vi "SIMCOMCommunicationTool.vi"(4 "Slot":T1, 6 "Debug":bool=TRUE, 7 "MEID":string, 8 "error in":errorcluster, 9 "DelayTime":u32=100, 10 "通信协议名称":string, 11 "VISA资源名称":refnum<visa-resource-name>="COM26") -> (0 "error out":errorcluster, 1 "ReturnData":string, 2 "反馈结果":bool=TRUE, 3 "字符串数值":bool=TRUE, 5 "CMD":string="发送 重启:AT+CRESET\r反馈:\r\nOK\r\n\r\n")   [LabVIEW 2013]
doc: "本范例根据用户指示，对串口执行读写操作。范例运行时可按下“写入”或“读取”按钮，以及修改“读数”。\n\n设置的串口参数必须匹配连接仪器或设备的参数。本范例中，“读数”参数可指定串口读取的字节数。如端口字节超过指定的字节数，超出部分将不会被读取。如端口字节数少于指定的字节数，将返回超时错误。\n\n本范例可扩展流控制选项以包括XON和XOFF，从而允许用户选择控制字符。同时，用户可启用或禁用中止符。部分设备需要通过终止符确定命令字符串的结束位置。部分设备将发送终止符以说明待读取数据的末端。本范例演示了缓冲区中检测到终止符时，结束“读取”操作或添加终止符至“写入”数据末端的方法。"
uses:
  SystemCode/SysControl/Slot.ctl
  <vilib>/Utility/NIReport.llb/NI_report.lvclass
  C:/Program Files/National Instruments/LabVIEW 2013/examples/Instrument IO/Serial/support/Serial - Settings.ctl
  SourceCode/GlobalValue.vi
  <vilib>/Utility/error.llb/Error Cluster From Error Code.vi
  <vilib>/addons/_office/excel.llb/Excel Get Data ([str]).vi
  <vilib>/Instr/_visa.llb/VISA Configure Serial Port (Instr).vi
  <vilib>/ErrorRing/Error Ring.xnode
  <vilib>/addons/_office/NI_ReportGenerationToolkit.lvlib
  <vilib>/Utility/NIReport.llb/Excel/NI_Excel.lvclass
panel:
  out "Data":string[][](array[string])=[["8986031490021881534", "460036161669975", "2A645416CB435F94", "8006A127", "460036161669975@mycdma.cn", "DB60264368A1D188", "18101891253", "A1000021A59070"], ["8986031490021881535", "460036161669976", "32FA5764D69C76BE", "80FAE4E6", "460036161669976@mycdma.cn", "B3AA1B3D2F0D5593", "18964872399", "A1000021A58D61"], ["", "", "", "", "", "", "", ""], ["", "", "", "", "", "", "", ""], ["", "", "", "", "", "", "", ""], ["", "", "", "", "", "", "", ""], ["", "", "", "", "", "", "", ""], ["", "", "", "", "", "", "", ""], ["", "", "", "", "", "", "", ""], ["", "", "", "", "", "", "", ""], ["", "各位，模块烧号主要是写五码，包括IMSI、AKEY、MEID（ESN）、AN(EVDO USER)、AAA(EVDO PWD)。", "", "", "", "", "", ""], ["", "其中ESN和MEID在模块出厂时已经写入，两者均可通过AT指令读取，但ESN不可更改。", "", "", "", "", "", ""], ["", "经询问及实际测试，上海电信绑定ESN号而广东电信未绑定，意味着上海电信五码烧录到其它模块是不可用的，但广东电信则无此限制。", "", "", "", "", "", ""], ["", "", "", "", "", "", "", ""], ["", "", "", "", "", "", "", ""], ["", "目前已确定跟上海电信合作，后续模块及卡号使用过程中，如遇到模块损坏，则意味着该卡必须销号（除非向电信申请绑定新的ESN），否则烧录到其它模块中是没用的。", "", "", "", "", "", ""]]
  in  "命令列表":u16(ring)=18 items=["查询RTRECF", "设置RTRECF", "查询MEID", "设置MEID", "查询ESN", "设置ESN", "查询AKEY", "设置AKEY", "查询IMSI1", "设置IMSI1", "查询IMSI2", "设置IMSI2", "查询IMSI3", "设置IMSI3", "设置EVDO账号", "设置EVDO密码", "打开音频LOOPBACK", "关闭音频LOOPBACK", "重启", "打开网络", "查询网络状态", "连网测试", "查询CIP", "切换声音通道", "测试登录", "拨号", "挂断", "查询IP", "AT+CSOCKAUTHNV", "AT+CSOCKAUTH", "查询2G信号", "查询3G信号", "H330测试通讯", "H330打开音频回环", "H330关闭音频回环", "H330拨号"]
  out "ConfigPath":string="D:\\导航\\T-BOX\\新建文件夹\\config\\通信协议.xls"
  out "DataType":string="AT+CRESET"
  out "命令":string="AT+CRESET\r"
  out "响应":string="\r\nOK\r\n"
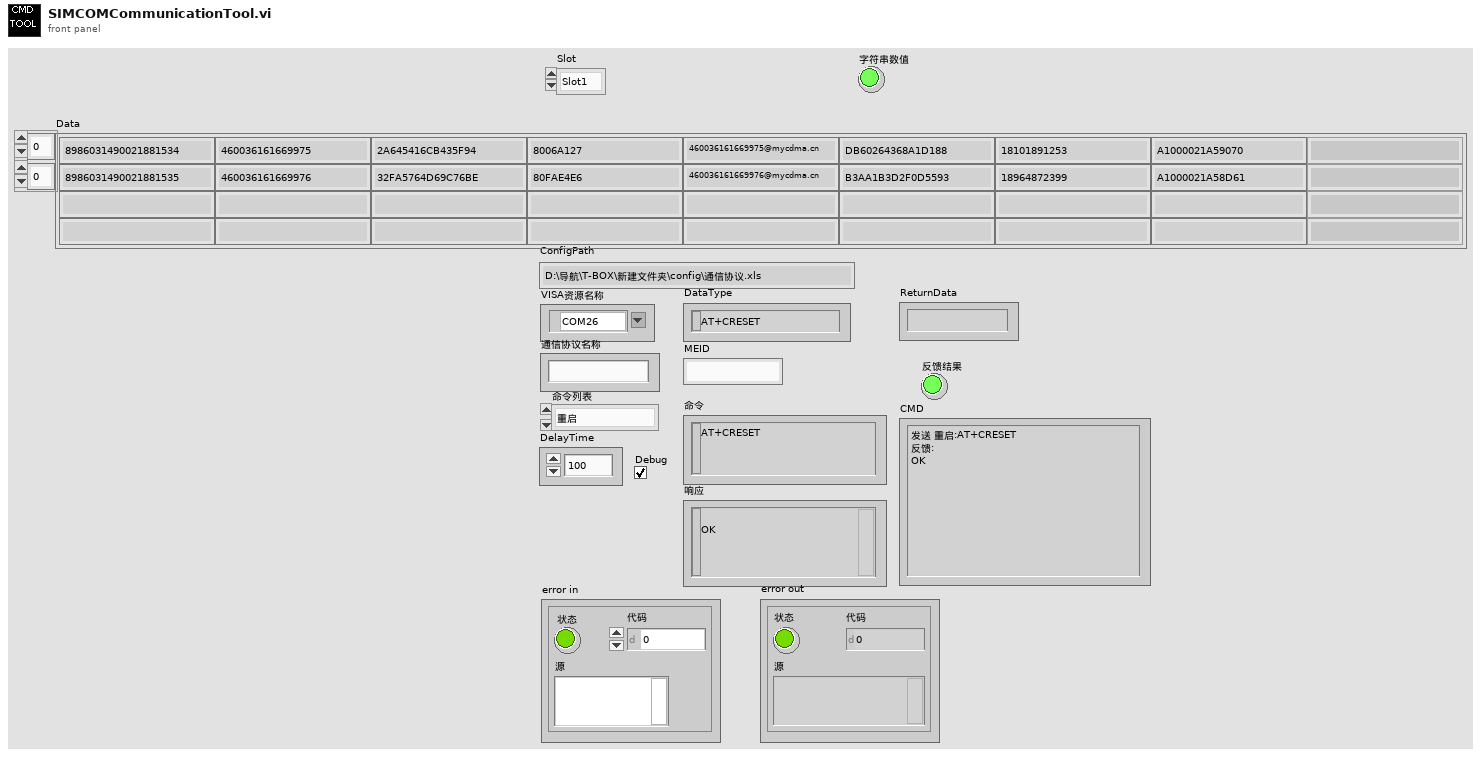
[diagram p1: front panel]
types:
  T1 = typedef "Slot.ctl" = enum16{"Slot1", "Slot2", "Slot3", "Slot4"}
  T2 = enum32{"invalid app kind", "Development System", "Run Time System", "Student Edition", "Embedded LabVIEW", "Evaluation", "Custom"}
  T3 = enum16{"maximized", "minimized", "normal", "no change"}
  T4 = enum16{"Standard Report", "HTML", "Word", "Excel"}
  T5 = typedef "Serial - Settings.ctl" = cluster{"波特率":u32, "数据比特":u16, "奇偶":enum16{"None", "Odd", "Even", "Mark", "Space"}, "停止位":u16, "流控制":u16}
  T6 = cluster{"IMSI":string, "AKEY":string, "ESN":string, "EVDO账号":string, "EVDO密码":string, "设备号":string}
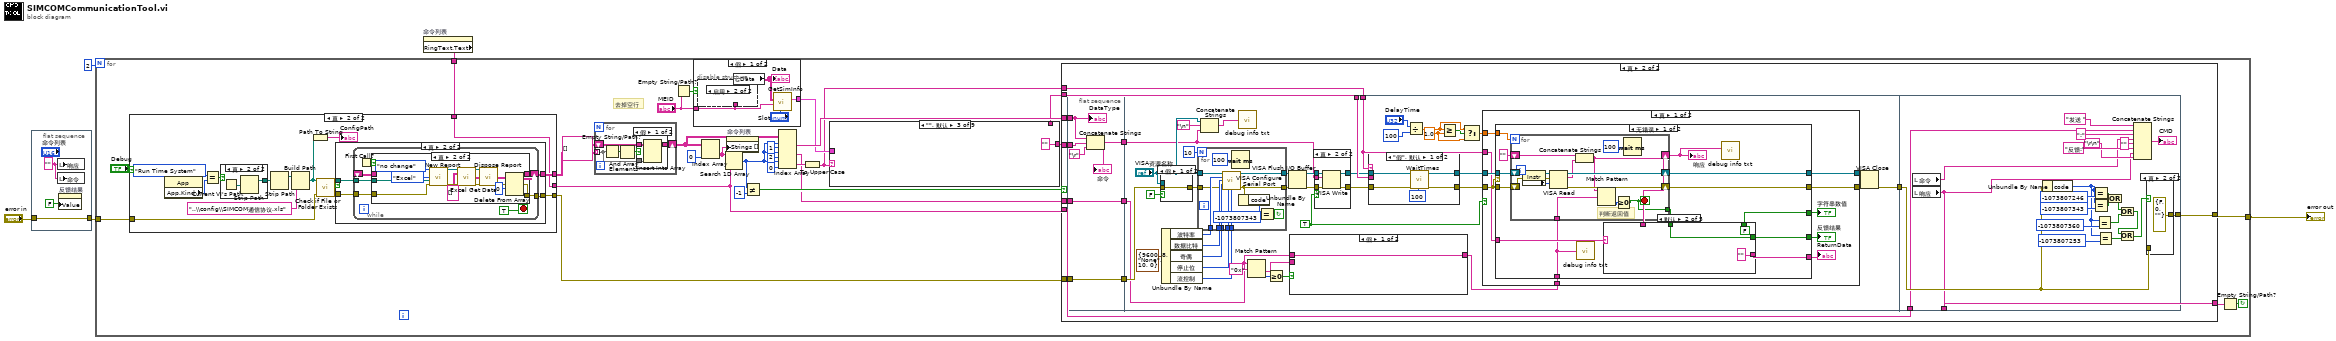
[diagram p0: block diagram]
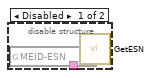
[diagram p2: hidden frame]
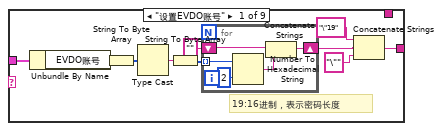
[diagram p5: hidden frame]
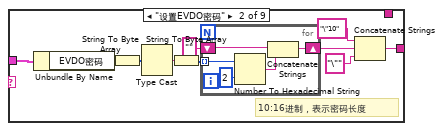
[diagram p6: hidden frame]
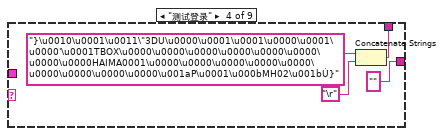
[diagram p7: hidden frame]
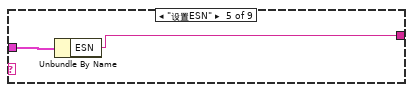
[diagram p8: hidden frame]
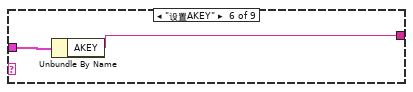
[diagram p9: hidden frame]
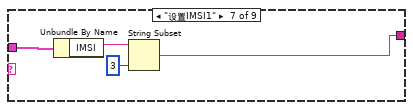
[diagram p10: hidden frame]
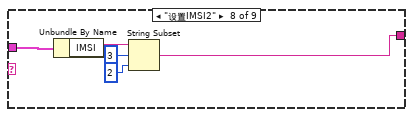
[diagram p11: hidden frame]
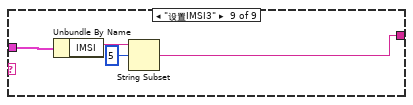
[diagram p12: hidden frame]
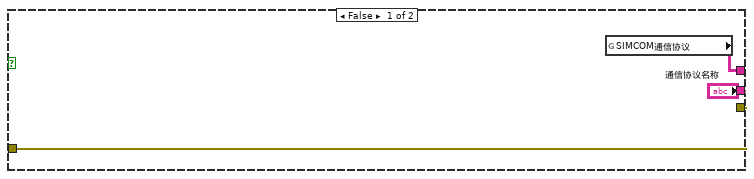
[diagram p13: hidden frame]
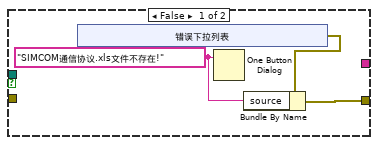
[diagram p14: hidden frame]
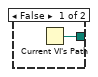
[diagram p16: hidden frame]
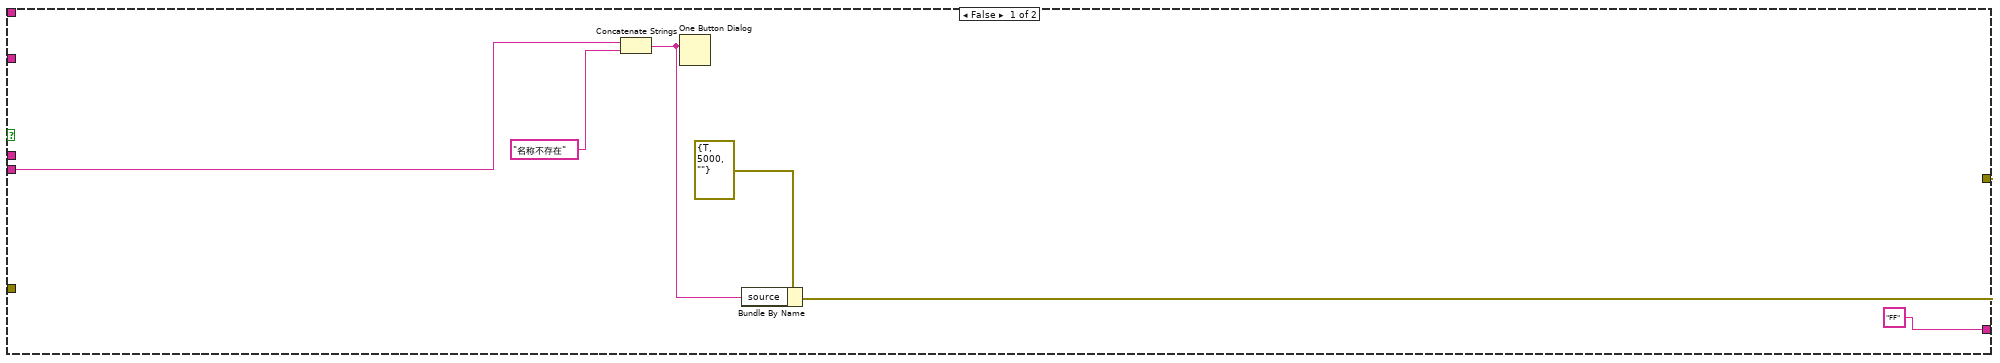
[diagram p17: hidden frame]
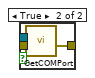
[diagram p18: hidden frame]
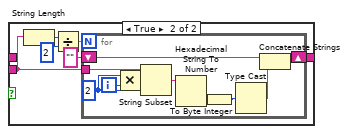
[diagram p19: hidden frame]
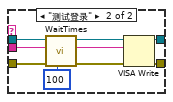
[diagram p20: hidden frame]
diagram:
  n1 = flat-sequence {
    tunnel: "error in" -> [w7]
    tunnel: [w7] -> w2
    frame #0 {
      w8 = "" ("响应")
      n2 = local write "响应"(w8) -> ()
      n3 = local write "命令"(w8) -> ()
      n4 = property on="反馈结果" class="Bool (严格)"("Value"=FALSE ("反馈结果")) -> ()  [unwired: 2 in, 2 out]
    }
  }
  n5 = property on="命令列表" class="Ring (严格)"() -> ("RingText.Text"=w1:string)  [unwired: 2 in, 2 out]
  n6 = for {
    N: 2 -> [_]
    tunnel: w2 -> [w24]
    tunnel: [w36] -> w5
    tunnel: w1 -> [w17]
    stop <- w22 continue-if-true
    # "去掉空行"
    n7 = case shown="真" "Debug" {
      tunnel: [w105 w110] -> w35
      tunnel: w24 -> [w105 w109]
      tunnel: ["通信协议名称" w107] -> w28
      tunnel: [w104 w108] -> w19
      tunnel: w17 -> [_ w107]
      frame False {
        n8 = global read "GlobalValue.vi" "SIMCOM通信协议"() -> (w104:string[][])
      }
      frame True {
        n9 = property class="App"() -> ("App.Kind"=w119:T2)  [unwired: 2 in, 2 out]
        n10 = Equal?(x=T2."Run Time System" ("y"), y=w119) -> (x = y?=w121:bool)
        n11 = case shown="真" w121 {
          tunnel: [w155 w157] -> w120
          frame False {
            n12 = Current VI's Path() -> (path=w155:path)
          }
          frame True {
            n13 = Current VI's Path() -> (path=w156:path)
            n14 = Strip Path(path=w156) -> (stripped path=w157:path)  [unwired: 1 out]
          }
        }
        n15 = Strip Path(path=w120) -> (stripped path=w114:path)  [unwired: 1 out]
        n16 = Build Path(base path=w114, name or relative path="..\\config\\SIMCOM通信协议.xls" ("连接的字符串")) -> (appended path=w116:path)
        n17 = Path To String(path=w116) -> (string=→"ConfigPath":string)
        n18 = call <vilib>:"Check if File or Folder Exists.vi"("error in (no error)"=w109, "path"=w116) -> ("error out"=w111:errorcluster, "file or folder exists?"=w113:bool, "dup path"=w112:path)  [unwired: 7 out]
        n19 = case shown="真" w113 {
          tunnel: w112 -> [_ w132]
          tunnel: w111 -> [_ w131]
          tunnel: [w123 w130] -> w110
          tunnel: [_ w129] -> w108
          frame False {
            w124 = "SIMCOM通信协议.xls文件不存在!" ("消息")
            n20 = xnode "错误下拉列表"() -> ("错误输出"=w122:errorcluster)
            n21 = One Button Dialog(message=w124) -> ()  [unwired: 1 in, 1 out]
            n22 = Bundle By Name(cluster=w122, "source"=w124) -> (w123:errorcluster)
          }
          frame True {
            n23 = while {
              tunnel: w132 -> [w138]
              tunnel: [w137] -> w130
              tunnel: w131 -> [w136]
              shift-right: [w139] -> w129
              shift-left: _ -> [w134]
              stop <- TRUE stop-if-true
              n24 = First Call?() -> (First Call?: T/F=w133:bool)
              n25 = case shown="真" w133 {
                tunnel: [w141 w145] -> w139
                tunnel: w138 -> [_ w144]
                tunnel: [w140 w143] -> w137
                tunnel: w136 -> [w140 w142]
                tunnel: w134 -> [w141 _]
                frame False {
                }
                frame True {
                  n26 = call <vilib>:"New Report.vi"("window state (normal)"=T3."no change", "report type"=T4."Excel", "template (empty)"=w144, "error in (no error)"=w142) -> ("report out"=w150:refnum<class "NI_report.lvclass">, "error out"=w151:errorcluster)  [unwired: 2 in, 8 out]
                  n27 = call-poly <vilib>:"Excel Get Data.vi"("report in"=w150, "data type"=string[][] [], "error in (no error)"=w151) -> ("report out"=w147:refnum<class "NI_report.lvclass">, "data"=w152:string[][], "error out"=w146:errorcluster)  [unwired: 10 in]
                  n28 = call-dynamic "Dispose Report.vi"("report in"=w147, "error in (no error)"=w146) -> ("error out"=w143:errorcluster)  [unwired: 3 in, 10 out]
                  n29 = Delete From Array(array=w152, index (row)=0 ("索引 (行)")) -> (array with subset deleted=w145:string[][])  [unwired: 2 in, 1 out]
                }
              }
            }
          }
        }
      }
    }
    n30 = for {
      tunnel: w19 -> [w43] mode=indexing
      shift-right: [w46] -> w18
      shift-left: string[][] [] -> [w47]
      n31 = Empty String/Path?(string/path=w43) -> (empty?=w45:bool[])
      n32 = And Array Elements(Boolean array=w45) -> (logical AND=w44:bool)
      n33 = case shown="假" w44 {
        tunnel: w47 -> [w50 w51]
        tunnel: [w49 w51] -> w46
        tunnel: w43 -> [w48 _]
        frame False {
          n34 = Insert Into Array(array=w50, new element=w48) -> (w49:string[][])  [unwired: 2 in]
        }
        frame True {
        }
      }
    }
    n35 = Empty String/Path?(string/path="MEID") -> (empty?=w10:bool)
    n36 = case shown="假" w10 {
      tunnel: [w40 _] -> w14
      tunnel: "MEID" -> [w37 _]
      frame False {
        n37 = disable-structure shown="启用" {
          disable-tunnel: w37 -> [w41 _]
          frame Disabled {
            n38 = global read "GlobalValue.vi" "MEID-ESN"() -> (w42:string[][])
            n39 = call "GetESN.vi"("MEID"=w41, "Data"=w42) -> ()  [unwired: 9 in, 1 out]
          }
          frame Enabled {
          }
        }
        n40 = global read "GlobalValue.vi" "Data"() -> (w39:string[][])
        "Data" <- w39
        n41 = call "GetSimInfo.vi"("Slot"="Slot", "MEID"=w37, "Data"=w39) -> ("SIMInfo"=w40:T6)  [unwired: 6 in, 2 out]
      }
      frame True {
      }
    }
    n42 = Index Array(array=w18, index (col)=0 ("禁用的索引 (列)")) -> (element=w26:string[])  [unwired: 1 in]
    n43 = Search 1D Array(1D array=w26, element=w28) -> (index of element=w21:i32)  [unwired: 1 in]
    n44 = property on="命令列表" class="Ring (严格)"("Strings []"=w26) -> ()  [unwired: 2 in, 2 out]
    n45 = Not Equal?(x=w21, y=-1) -> (x != y?=w30:bool)
    n46 = Index Array(array=w18, index (row) #1=w21, index (col) #1=1 ("索引 (列)"), index (row) #2=w21, index (col) #2=2 ("索引 (列)"), index (row) #3=w21, index (col) #3=0 ("索引 (列)")) -> (element #1=w15:string, element #2=w11:string, element #3=w16:string)
    n47 = To Upper Case(1:w16) -> (0:w12:string)
    n48 = case shown="\"\", 默认" w12 {
      tunnel: [w54 w69 "" "" ("IMSI") w87 w89 w91 w96 w101] -> w29
      tunnel: w14 -> [w53 w67 _ _ w88 w90 w94 w99 w103]
      tunnel: [_ _ _ w83 _ _ _ _ _] -> w13
      frame "设置EVDO账号" {
        # "19:16进制，表示密码长度"
        n49 = Unbundle By Name(w53) -> ("EVDO账号"=w52:string)
        n50 = String To Byte Array(string=w52) -> (unsigned byte array=w61:u8[])
        n51 = Type Cast(x=w61) -> (*(type *) &x=w59:string)  [unwired: 1 in]
        n52 = String To Byte Array(string=w59) -> (unsigned byte array=w60:u8[])
        n53 = for {
          tunnel: w60 -> [w66] mode=indexing
          shift-right: [w64] -> w55
          shift-left: "" -> [w63]
          n54 = Number To Hexadecimal String(1:i16 2 ("宽度(-)"), 2:w66) -> (0:w65:string)
          n55 = Concatenate Strings(w63, w65) -> (w64:string)
        }
        n56 = Concatenate Strings("\"19" ("字符串"), w55, "\"" ("字符串")) -> (w54:string)
      }
      frame "设置EVDO密码" {
        # "10:16进制，表示密码长度"
        n57 = Unbundle By Name(w67) -> ("EVDO密码"=w68:string)
        n58 = String To Byte Array(string=w68) -> (unsigned byte array=w76:u8[])
        n59 = Type Cast(x=w76) -> (*(type *) &x=w74:string)  [unwired: 1 in]
        n60 = String To Byte Array(string=w74) -> (unsigned byte array=w75:u8[])
        n61 = for {
          tunnel: w75 -> [w81] mode=indexing
          shift-right: [w79] -> w72
          shift-left: "" -> [w78]
          n62 = Number To Hexadecimal String(1:i16 2 ("宽度(-)"), 2:w81) -> (0:w80:string)
          n63 = Concatenate Strings(w78, w80) -> (w79:string)
        }
        n64 = Concatenate Strings("\"10" ("字符串"), w72, "\"" ("字符串")) -> (w69:string)
      }
      frame "", Default {
      }
      frame "测试登录" {
        n65 = Concatenate Strings("}\u0010\u0001\u0011\"3DU\u0000\u0001\u0001\u0000\u0001\u0000'\u0001TBOX\u0000\u0000\u0000\u0000\u0000\u0000\u0000\u0000HAIMA0001\u0000\u0000\u0000\u0000\u0000\u0000\u0000\u0000\u0000\u001aP\u0001\u000bMH02\u001bÚ}" ("字符串"), "\r") -> (w83:string)
      }
      frame "设置ESN" {
        n66 = Unbundle By Name(w88) -> ("ESN"=w87:string)
      }
      frame "设置AKEY" {
        n67 = Unbundle By Name(w90) -> ("AKEY"=w89:string)
      }
      frame "设置IMSI1" {
        n68 = Unbundle By Name(w94) -> ("IMSI"=w93:string)
        n69 = String Subset(string=w93, length (rest)=3 ("长度（剩余）")) -> (substring=w91:string)  [unwired: 1 in]
      }
      frame "设置IMSI2" {
        n70 = Unbundle By Name(w99) -> ("IMSI"=w98:string)
        n71 = String Subset(string=w98, offset (0)=3 ("偏移量(0)"), length (rest)=2 ("长度（剩余）")) -> (substring=w96:string)
      }
      frame "设置IMSI3" {
        n72 = Unbundle By Name(w103) -> ("IMSI"=w102:string)
        n73 = String Subset(string=w102, offset (0)=5 ("偏移量(0)")) -> (substring=w101:string)  [unwired: 1 in]
      }
    }
    n74 = case shown="真" w30 {
      tunnel: w28 -> [w163 w168]
      tunnel: w15 -> [_ w176]
      tunnel: w29 -> [_ w175]
      tunnel: w35 -> [_ w174]
      tunnel: [w159 w172] -> w36
      tunnel: ["FF" ("响应") w170] -> w23
      tunnel: w13 -> [_ w167]
      tunnel: w12 -> [_ w166]
      tunnel: w11 -> [_ w165]
      frame False {
        n75 = Concatenate Strings(w163, "名称不存在" ("消息")) -> (w160:string)
        n76 = One Button Dialog(message=w160) -> ()  [unwired: 1 in, 1 out]
        n77 = Bundle By Name(cluster=errorcluster {"status"=TRUE, "code"=5000, "source"=""} ("error in 1 (no error)"), "source"=w160) -> (w159:errorcluster)
      }
      frame True {
        n78 = flat-sequence {
          tunnel: w176 -> [w181]
          tunnel: w175 -> [w180]
          tunnel: w174 -> [w182]
          tunnel: [w182] -> w173
          tunnel: [w179] -> w169
          tunnel: w165 -> [w177]
          tunnel: [w177] -> w164
          tunnel: w173 -> [w206]
          tunnel: [w214] -> w171
          tunnel: w169 -> [w185]
          tunnel: w167 -> [w208]
          tunnel: w166 -> [w207]
          tunnel: w164 -> [w189]
          tunnel: [w373] -> w172
          tunnel: w171 -> [w372]
          tunnel: w168 -> [w369]
          tunnel: [w363] -> w170
          frame #0 {
            n79 = Concatenate Strings(w181, w180, "\r") -> (w179:string)
            "命令" <- w179
            "DataType" <- w181
          }
          frame #1 {
            w202 = 1.0 ("y")
            w209 = TRUE
            n80 = case shown="假" FALSE {
              tunnel: w206 -> [w223 w226]
              tunnel: [w223 w225] -> w205
              tunnel: "VISA资源名称" -> [_ w224]
              frame False {
              }
              frame True {
                n81 = call "GetCOMPort.vi"("错误输入（无错误）"=w226, "VISA引用句柄输入"=w224) -> ("错误输出"=w225:errorcluster)  [unwired: 8 in, 1 out]
              }
            }
            n82 = Unbundle By Name(T5 {"波特率"=9600, "数据比特"=8, "奇偶"=enum."None", "停止位"=10, "流控制"=0} ("串口设置")) -> ("波特率"=w219:u32, "数据比特"=w220:u16, "奇偶"=w221:enum16{"None", "Odd", "Even", "Mark", "Space"}, "停止位"=w222:u16, "流控制"=w215:u16)
            n83 = for {
              N: 10 -> [_]
              tunnel: w222 -> [w256]
              tunnel: w221 -> [w255]
              tunnel: w220 -> [w254]
              tunnel: w219 -> [w253]
              tunnel: w215 -> [w252]
              tunnel: [w245] -> w213
              tunnel: [w244] -> w212
              tunnel: "VISA资源名称" -> [w251]
              tunnel: w205 -> [w250]
              stop <- w246 continue-if-true
              n84 = call-poly "VISA Configure Serial Port"("VISA resource name"=w251, "baud rate (9600)"=w253, "data bits (8)"=w254, "parity (0:none)"=w255, "error in (no error)"=w250, "stop bits (10: 1 bit)"=w256, "flow control (0:none)"=w252) -> ("VISA resource name out"=w244:refnum<visa-resource-name>, "error out"=w245:errorcluster)  [unwired: 3 in, 4 out]
              n85 = Wait (ms)(milliseconds to wait=u32 100 ("等待时间（毫秒）")) -> ()  [unwired: 1 out]
              n86 = Unbundle By Name(w245) -> ("code"=w248:i32)
              n87 = Equal?(x=w248, y=-1073807343) -> (x = y?=w246:bool)
            }
            n88 = Concatenate Strings("VISA资源名称", "\n", w185) -> (w184:string)
            n89 = call "debug info txt.vi"("data"=w184) -> ()  [unwired: 7 in]
            n90 = Match Pattern(string=w189, regular expression="0x" ("正则表达式")) -> (after substring=w191:string, offset past match=w192:i32)  [unwired: 1 in, 2 out]
            n91 = Greater Or Equal To 0?(x=w192) -> (x >= 0?=w190:bool)
            n92 = VISA Flush I/O Buffer(VISA resource name=w212, error in (no error)=w213) -> (VISA resource name out=w211:refnum<visa-resource-name>, error out=w210:errorcluster)  [unwired: 1 in]
            n93 = case shown="假" w190 {
              tunnel: w191 -> [_ w229]
              tunnel: [w227 w228] -> w188
              tunnel: w189 -> [w227 _]
              frame False {
              }
              frame True {
                n94 = String Length(string=w229) -> (length=w232:i32)
                n95 = Divide(x=w232, y=2) -> (x/y=w230:dbl)
                n96 = for {
                  N: w230 -> [_]
                  tunnel: w229 -> [w238]
                  shift-right: [w240] -> w228
                  shift-left: "" -> [w239]
                  i -> [w236]
                  w234 = 2 ("x")
                  n97 = Multiply(x=w234, y=w236) -> (x*y=w235:i32)
                  n98 = String Subset(string=w238, offset (0)=w235, length (rest)=w234) -> (substring=w237:string)
                  n99 = Hexadecimal String To Number(string=w237) -> (number=w243:u32)  [unwired: 2 in, 1 out]
                  n100 = To Byte Integer(number=w243) -> (8bit integer=w242:i8)
                  n101 = Type Cast(x=w242) -> (*(type *) &x=w241:string)  [unwired: 1 in]
                  n102 = Concatenate Strings(w239, w241) -> (w240:string)
                }
              }
            }
            n103 = case shown="真" w209 {
              tunnel: w211 -> [w269 w274]
              tunnel: [w269 w273] -> w204
              tunnel: [w268 w272] -> w203
              tunnel: w210 -> [w268 w271]
              tunnel: w185 -> [_ w270]
              frame False {
              }
              frame True {
                n104 = VISA Write(VISA resource name=w274, write buffer=w270, error in (no error)=w271) -> (VISA resource name out=w273:refnum<visa-resource-name>, error out=w272:errorcluster)  [unwired: 1 out]
              }
            }
            n105 = case shown="\"假\", 默认" w207 {
              tunnel: w204 -> [w260 w267]
              tunnel: [w260 w266] -> w196
              tunnel: [w257 w265] -> w195
              tunnel: w203 -> [w258 w263]
              tunnel: w208 -> [_ w264]
              frame "假", Default {
                n106 = call "WaitTimes.vi"("WaitTimes"=u32 100, "error in (no error)"=w258) -> ("error out"=w257:errorcluster)  [unwired: 9 in]
              }
              frame "测试登录" {
                n107 = call "WaitTimes.vi"("WaitTimes"=u32 100, "error in (no error)"=w263) -> ("error out"=w262:errorcluster)  [unwired: 9 in]
                n108 = VISA Write(VISA resource name=w267, write buffer=w264, error in (no error)=w262) -> (VISA resource name out=w266:refnum<visa-resource-name>, error out=w265:errorcluster)  [unwired: 1 out]
              }
            }
            n109 = Divide(x="DelayTime", y=u32 100) -> (x/y=w201:dbl)
            n110 = Greater Or Equal?(x=w201, y=w202) -> (x >= y?=w200:bool)
            n111 = Select(t=w201, s=w200, f=w202) -> (s? t:f=w198:dbl)
            n112 = case shown="真" w209 {
              tunnel: [w283 w356] -> w216
              tunnel: w196 -> [w282 w356]
              tunnel: [w284 w355] -> w217
              tunnel: w195 -> [w280 w355]
              tunnel: w207 -> [w281 _]
              tunnel: w198 -> [w279 _]
              tunnel: w188 -> [w278 _]
              frame True {
                n113 = case shown="无错误" w280 {
                  tunnel: [w297 w354] -> w284
                  tunnel: [w296 w353] -> w283
                  tunnel: w282 -> [w295 w353]
                  tunnel: w280 -> [w294 w354]
                  tunnel: w281 -> [w291 _]
                  tunnel: w279 -> [w292 _]
                  tunnel: w278 -> [w285 _]
                  tunnel: [w289 "" ("read buffer")] -> w277
                  tunnel: [w288 w351] -> w276
                  tunnel: [w287 w351] -> w275
                  frame No Error {
                    n114 = for {
                      N: w292 -> [_]
                      shift-right: [w350] -> w297
                      shift-left: w294 -> [w344]
                      shift-right: [w339] -> w286
                      shift-left: "" ("read buffer") -> [w343]
                      shift-right: [w349] -> w296
                      shift-left: w295 -> [w345]
                      tunnel: w285 -> [w338]
                      tunnel: [w337] -> w290
                      stop <- w337 stop-if-true
                      # "判断返回值"
                      n115 = property class="Instr"(reference=w345, error in=w344) -> (reference out=w348:refnum<visa-resource-name>, error out=w347:errorcluster, "Serial Settings:Number of Bytes at Serial Port"=w346:u32)
                      n116 = VISA Read(VISA resource name=w348, byte count=w346, error in (no error)=w347) -> (VISA resource name out=w349:refnum<visa-resource-name>, read buffer=w341:string, error out=w350:errorcluster)  [unwired: 1 out]
                      n117 = Concatenate Strings(w343, w341) -> (w339:string)
                      n118 = Match Pattern(string=w339, regular expression=w338) -> (offset past match=w342:i32)  [unwired: 1 in, 3 out]
                      n119 = Greater Or Equal To 0?(x=w342) -> (x >= 0?=w337:bool)
                      n120 = Wait (ms)(milliseconds to wait=u32 100 ("等待时间（毫秒）")) -> ()  [unwired: 1 out]
                    }
                    "响应" <- w286
                    n121 = call "debug info txt.vi"("data"=w285) -> ()  [unwired: 7 in]
                    n122 = case shown="默认" w291 {
                      tunnel: [w301 "" ("read buffer") w318 w324 w331] -> w289
                      tunnel: w286 -> [w306 _ w319 w327 w334]
                      tunnel: w290 -> [w300 w311 w315 _ _]
                      tunnel: [w299 w311 w313 FALSE FALSE] -> w288
                      tunnel: [FALSE FALSE FALSE TRUE TRUE] -> w287
                      frame "查询ESN" {
                        n123 = Match Pattern(string=w306, regular expression="+ESN: " ("正则表达式")) -> (after substring=w308:string)  [unwired: 1 in, 3 out]
                        n124 = Match Pattern(string=w308, regular expression="\r\n\r\nOK" ("正则表达式")) -> (before substring=w301:string)  [unwired: 1 in, 3 out]
                        n125 = String Length(string=w301) -> (length=w304:i32)
                        n126 = Greater?(x=w304, y=1) -> (0:w302:bool)
                        n127 = And(x=w300, y=w302) -> (x .and. y?=w299:bool)
                      }
                      frame Default {
                      }
                      frame "查询MEID" {
                        n128 = Match Pattern(string=w319, regular expression="+SMEID: " ("正则表达式")) -> (after substring=w322:string)  [unwired: 1 in, 3 out]
                        n129 = Match Pattern(string=w322, regular expression="\r\n\r\nOK" ("正则表达式")) -> (before substring=w318:string)  [unwired: 1 in, 3 out]
                        n130 = String Length(string=w318) -> (length=w317:i32)
                        n131 = Greater?(x=w317, y=1) -> (0:w314:bool)
                        n132 = And(x=w315, y=w314) -> (x .and. y?=w313:bool)
                      }
                      frame "查询2G信号" {
                        n133 = Match Pattern(string=w327, regular expression="+CSQ: " ("正则表达式")) -> (after substring=w329:string)  [unwired: 1 in, 3 out]
                        n134 = Match Pattern(string=w329, regular expression="[0-9]+" ("正则表达式")) -> (match substring=w324:string)  [unwired: 1 in, 3 out]
                      }
                      frame "查询3G信号" {
                        n135 = Match Pattern(string=w334, regular expression="HDRCSQ: " ("正则表达式")) -> (after substring=w336:string)  [unwired: 1 in, 3 out]
                        n136 = Match Pattern(string=w336, regular expression="\r\n\r\nOK" ("正则表达式")) -> (before substring=w331:string)  [unwired: 1 in, 3 out]
                      }
                    }
                    n137 = call "debug info txt.vi"("data"=w286) -> ()  [unwired: 7 in]
                  }
                  frame Error {
                    w351 = FALSE
                  }
                }
                "ReturnData" <- w277
                "反馈结果" <- w276
                "字符串数值" <- w275
              }
              frame False {
              }
            }
            n138 = VISA Close(VISA resource name=w216, error in (no error)=w217) -> (error out=w214:errorcluster)
          }
          frame #2 {
            n139 = local read "命令"() -> (w364:string)
            n140 = local read "响应"() -> (w363:string)
            n141 = Unbundle By Name(w372) -> ("code"=w361:i32)
            n142 = Equal?(x=w361, y=-1073807246) -> (x = y?=w370:bool)
            n143 = Equal?(x=w361, y=-1073807343) -> (x = y?=w367:bool)
            n144 = Equal?(x=w361, y=-1073807360) -> (x = y?=w365:bool)
            n145 = Equal?(x=w361, y=-1073807253) -> (x = y?=w358:bool)
            n146 = Or(x=w370, y=w367) -> (x .or. y?=w366:bool)
            n147 = Or(x=w366, y=w365) -> (x .or. y?=w359:bool)
            n148 = Or(x=w359, y=w358) -> (x .or. y?=w357:bool)
            n149 = Concatenate Strings("发送 " ("字符串"), w369, ":" ("字符串"), w364, "" ("字符串"), "反馈:" ("字符串"), w363, "\r\n") -> (→"CMD":string)
            n150 = case shown="真" w357 {
              tunnel: [w380 errorcluster {"status"=FALSE, "code"=0, "source"=""} ("t")] -> w373
              tunnel: w372 -> [w380 _]
              frame False {
              }
              frame True {
              }
            }
          }
        }
      }
    }
    n151 = Empty String/Path?(string/path=w23) -> (empty?=w22:bool)
  }
  "error out" <- w5
